vi "init data logging.vi"() -> (3 "output cluster":T1)   [LabVIEW 2025]
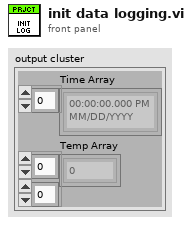
[diagram p1: front panel]
types:
  T1 = cluster{"Time Array":timestamp[], "Temp Array":dbl[][]}
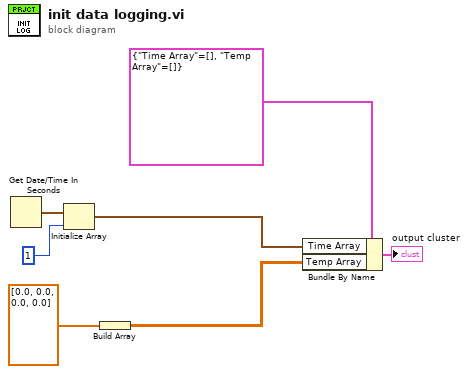
[diagram p0: block diagram]
diagram:
  n1 = Get Date/Time In Seconds() -> (seconds since 1Jan1904=w6:timestamp)
  n2 = Initialize Array(w6, 1 ("dimension size")) -> (w3:timestamp[])
  n3 = Build Array(dbl[] [0.0, 0.0, 0.0, 0.0]) -> (w2:dbl[][])
  n4 = Bundle By Name(cluster=T1 {"Time Array"=[], "Temp Array"=[]}, "Time Array"=w3, "Temp Array"=w2) -> (→"output cluster":T1)
